vi "Controls State (single).vi"(8 "error in":errorcluster, 10 "Disabled":T1(ring), 11 "Ctl Refnum":refnum<vi>) -> (0 "error out":errorcluster)   [LabVIEW 2020, in "Enum Queue State Machine.lvlib"]
uses:
  Enum Queue State Machine.lvlib
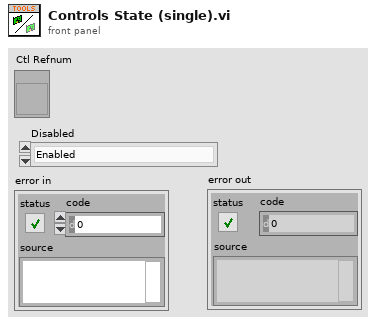
[diagram p1: front panel]
types:
  T1 = enum8{"Enabled", "Disabled", "Disabled and Grayed Out"}
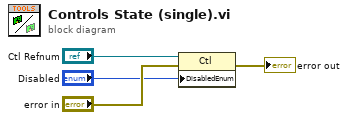
[diagram p0: block diagram]
diagram:
  n1 = property class="Ctl"(reference="Ctl Refnum", error in="error in", "DisabledEnum"="Disabled") -> (error out=→"error out":errorcluster)  [unwired: 1 out]
